vi "Get Logging Options.vi"(8 "error in (no error)":errorcluster, 11 "IoT Session in":refnum<class "IoT Session.lvclass">) -> (0 "error out":errorcluster, 1 "Role ARN":string, 2 "Log Level":string, 3 "IoT Session out":refnum<class "IoT Session.lvclass">, 4 "Role Name":string)   [LabVIEW 2015, in "NI_AWS_IoT.lvlib" / "IoT Session.lvclass"]
uses:
  IoT Session.lvclass
  Core/HTTP Request/Request Options.ctl
  Core/HTTP Request/Name Value Pair.ctl
  Core/HTTP Request/Region handling.ctl
  Core/HTTP Request/URL formatting.ctl
  Core/HTTP Request/HTTP Request.lvclass/HTTP Request.ctl
  Core/HTTP Request/Read Credentials.vi
  Core/HTTP Request/HTTP Request.lvclass
  JSON Parsing/NI_JSON Parsing.lvlib
  IAM/IAM Session/IAM Session.lvclass
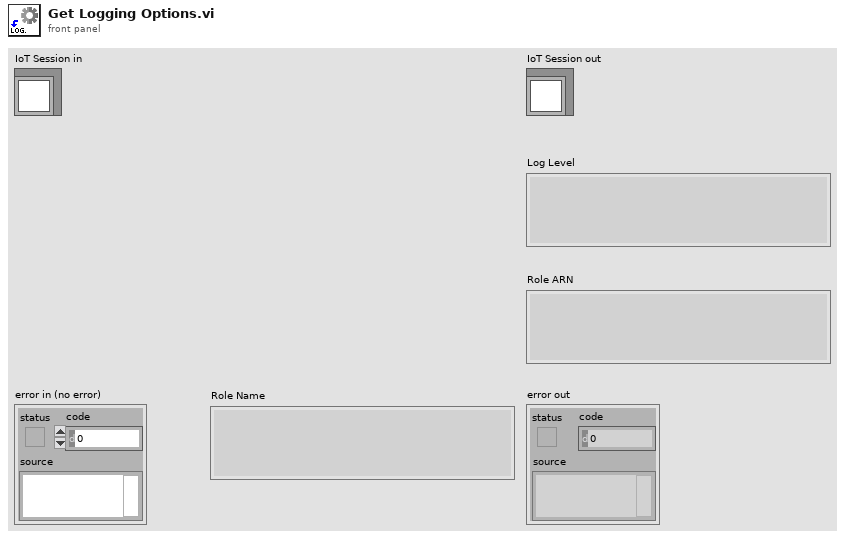
[diagram p1: front panel]
types:
  T1 = typedef "NI_AWS_Core.lvlib/HTTP Request.lvclass/Name Value Pair.ctl" = cluster{"name":string, "value":string}
  T2 = typedef "NI_AWS_Core.lvlib/HTTP Request.lvclass/Request Options.ctl" = cluster{"request headers":T1[], "request parameters":T1[], "request body":string, "region handling":T3, "URL formatting":T4}
  T3 = typedef "NI_AWS_Core.lvlib/HTTP Request.lvclass/Region handling.ctl" = enum16{"use region everywhere", "use region (authentication only)", "use region (URL only)", "ignore region everwhere"}
  T4 = typedef "NI_AWS_Core.lvlib/HTTP Request.lvclass/URL formatting.ctl" = enum16{"region-", "region."}
  T5 = typedef "NI_AWS_Core.lvlib/HTTP Request.lvclass/Response.ctl" = cluster{"Headers":string, "Body":string}
  T6 = typedef "NI_AWS_Core.lvlib/HTTP Request.lvclass/AWS Credentials.ctl" = cluster{"Access Key":string, "Secret Key":string}
  T7 = typedef "NI_AWS_IAM.lvlib/Role.ctl" = cluster{"Name":string, "ID":string, "Path":string, "ARN":string, "Policy Document":string, "Creation Date":string}
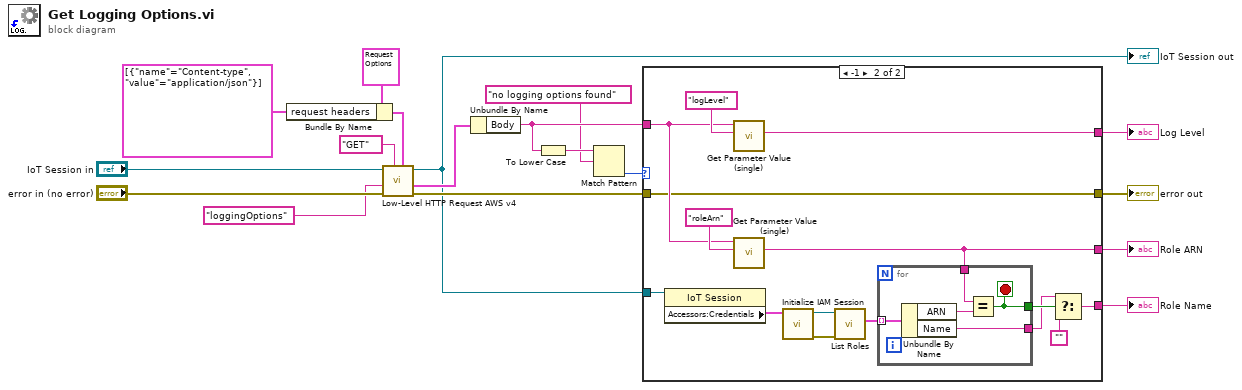
[diagram p0: block diagram]
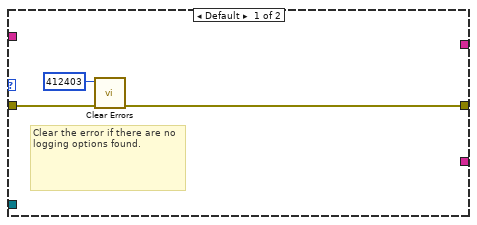
[diagram p2: hidden frame]
diagram:
  n1 = Bundle By Name(cluster=T2 {"request headers"=[], "request parameters"=[], "request body"="", "region handling"=enum."use region everywhere", "URL formatting"=enum."region."} ("Request Options"), "request headers"=T1[] [{"name"="Content-type", "value"="application/json"}]) -> (w14:T2)
  n2 = call "Low-Level HTTP Request AWS v4.vi"("Request Options"=w14, "HTTP-Verb"="GET", "error in (no error)"="error in (no error)", "URL Suffix"="loggingOptions" ("string"), "AWS Core in"="IoT Session in") -> ("error out"=w4:errorcluster, "Response"=w12:T5, "AWS Core out"=w2:refnum<class "IoT Session.lvclass">)  [unwired: 3 in, 1 out]
  "IoT Session out" <- w2
  n3 = Unbundle By Name(w12) -> ("Body"=w8:string)
  n4 = To Lower Case(string=w8) -> (all lower case string=w7:string)
  n5 = Match Pattern(string=w7, regular expression="no logging options found") -> (offset past match=w5:i32)  [unwired: 1 in, 3 out]
  n6 = case shown="-1" w5 {
    tunnel: [_ w35] -> w10
    tunnel: [_ w26] -> w9
    tunnel: w8 -> [_ w33]
    tunnel: w4 -> [w21 w32]
    tunnel: [w20 w32] -> w3
    tunnel: w2 -> [_ w31]
    tunnel: [_ w23] -> w1
    frame Default {
      # "Clear the error if there are no logging options found."
      n7 = call <vilib>:"Clear Errors.vi"("error in (no error)"=w21, "specific error code to clear (0: all)"=412403) -> ("error out"=w20:errorcluster)  [unwired: 4 in, 1 out]
    }
    frame -1 {
      n8 = property class="IoT Session"(reference=w31) -> ("Accessors:Credentials"=w30:T6)  [unwired: 1 in, 2 out]
      n9 = call "Get Parameter Value (single).vi"("Parameter Name"="logLevel", "JSON"=w33) -> ("Parameter Value"=w35:string)  [unwired: 6 in, 3 out]
      n10 = call "Get Parameter Value (single).vi"("Parameter Name"="roleArn", "JSON"=w33) -> ("Parameter Value"=w26:string)  [unwired: 6 in, 3 out]
      n11 = call "Initialize IAM Session.vi"("AWS Credentials"=w30) -> ("error out"=w28:errorcluster, "IAM Session"=w29:refnum<class "IAM Session.lvclass">)  [unwired: 9 in]
      n12 = call "List Roles.vi"("error in (no error)"=w28, "IAM Session in"=w29) -> ("Roles"=w27:T7[])  [unwired: 7 in, 2 out]
      n13 = for {
        tunnel: w27 -> [w41] mode=indexing
        tunnel: w26 -> [w39]
        tunnel: [w38] -> w25
        tunnel: [w37] -> w24
        stop <- w38 stop-if-true
        n14 = Unbundle By Name(w41) -> ("ARN"=w40:string, "Name"=w37:string)
        n15 = Equal?(x=w39, y=w40) -> (x = y?=w38:bool)
      }
      n16 = Select(t=w24, s=w25, f="") -> (s? t:f=w23:string)
    }
  }
  "error out" <- w3
  "Log Level" <- w10
  "Role ARN" <- w9
  "Role Name" <- w1
